vi "螺帽中心投影到槽平分线上-做一字槽中心.vi"(8 "Fitted Circle":T3, 9 "一字槽两边的角平分线":T2, 11 "Image In":T1) -> (1 "Radius (Pixels)":dbl, 3 "一字槽中心":cluster{"X":sgl, "Y":sgl})   [LabVIEW 2014]
uses:
  <vilib>/vision/Image Controls.llb/IMAQ Image.ctl
  <vilib>/vision/NI_Vision_Development_Module.lvlib
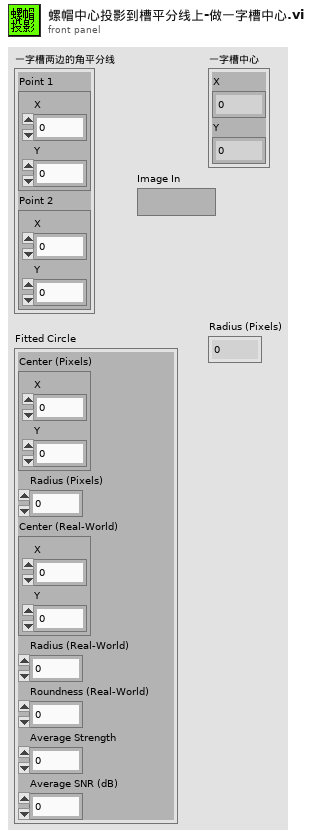
[diagram p1: front panel]
types:
  T1 = typedef "IMAQ Image.ctl" = refnum<image>
  T2 = cluster{"Point 1":cluster{"X":sgl, "Y":sgl}, "Point 2":cluster{"X":sgl, "Y":sgl}}
  T3 = cluster{"Center (Pixels)":cluster{"X":sgl, "Y":sgl}, "Radius (Pixels)":dbl, "Center (Real-World)":cluster{"X":sgl, "Y":sgl}, "Radius (Real-World)":dbl, "Roundness (Real-World)":dbl, "Average Strength":dbl, "Average SNR (dB)":dbl}
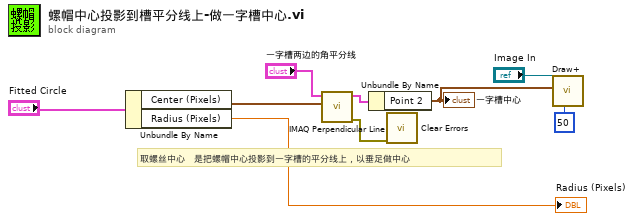
[diagram p0: block diagram]
diagram:
  # "取螺丝中心   是把螺帽中心投影到一字槽的平分线上，以垂足做中心"
  n1 = Unbundle By Name("Fitted Circle") -> ("Center (Pixels)"=w7:cluster{"X":sgl, "Y":sgl}, "Radius (Pixels)"=→"Radius (Pixels)":dbl)
  n2 = call "IMAQ Perpendicular Line"("Point"=w7, "Line"="一字槽两边的角平分线") -> ("error out"=w5:errorcluster, "Perpendicular Line"=w4:T2)  [unwired: 7 in, 1 out]
  n3 = Unbundle By Name(w4) -> ("Point 2"=w2:cluster{"X":sgl, "Y":sgl})
  "一字槽中心" <- w2
  n4 = call <vilib>:"Clear Errors.vi"("error in (no error)"=w5) -> ()  [unwired: 5 in, 2 out]
  n5 = call "Draw+.vi"("Width"=50, "input cluster"=w2, "Image In"="Image In") -> ()  [unwired: 3 in, 1 out]
